vi "set pixel clock.vi"(8 "error in (no error)":errorcluster, 11 "Thorcam in":refnum<class "Thorcam.lvclass">) -> (0 "error out":errorcluster, 3 "Thorcam out":refnum<class "Thorcam.lvclass">)   [LabVIEW 2012, in "Thorcam.lvclass"]
uses:
  Thorcam.lvclass
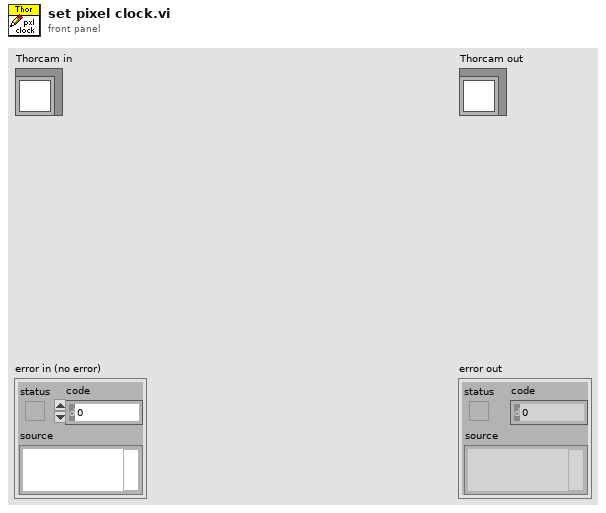
[diagram p1: front panel]
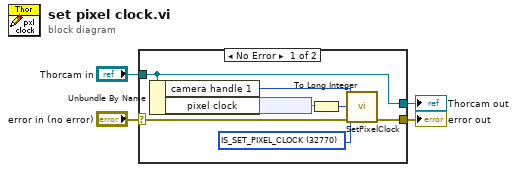
[diagram p0: block diagram]
diagram:
  n1 = case shown="No Error" "error in (no error)" {
    selector: "error in (no error)" -> [w12 w14]
    tunnel: [w11 w14] -> w3
    tunnel: [w5 w13] -> w1
    tunnel: "Thorcam in" -> [w5 w13]
    frame No Error {
      w9 = 32770 items=["IS_GET_PIXEL_CLOCK"=32768, "IS_GET_DEFAULT_PCLK"=32769, "IS_SET_PIXEL_CLOCK"=32770] ("Mode")
      n2 = Unbundle By Name(w5) -> ("camera handle 1"=w10:u32, "pixel clock"=w7:dbl[unit])
      n3 = node(w7) -> (w6:dbl)
      n4 = To Long Integer(number=w6) -> (32bit integer=w8:i32)
      n5 = call <instrlib>:"SetPixelClock.vi"("error in"=w12, "Mode"=w9, "Pixel Clock"=w8, "Camera Handle In"=w10) -> ("error out"=w11:errorcluster)  [unwired: 5 in, 2 out]
    }
    frame Error {
    }
  }
  "error out" <- w3
  "Thorcam out" <- w1
